vi "自定义DAC.vi"(8 "Vref V":dbl=2.56, 11 "数字编码":dbl[](array[numeric])) -> (2 "输出 V":dbl)   [LabVIEW 2020]
uses:
  <vilib>/express/express arith-compare/Formula/XNode/ExpressFormulaBlockNode.xnode
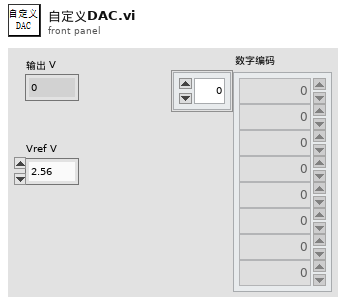
[diagram p1: front panel]
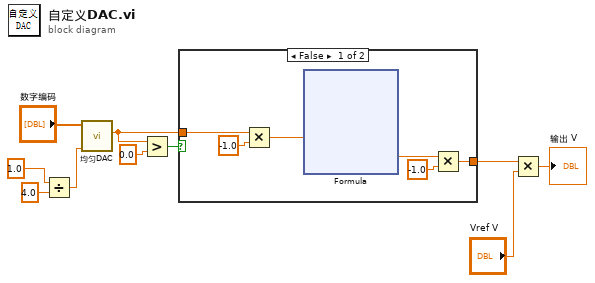
[diagram p0: block diagram]
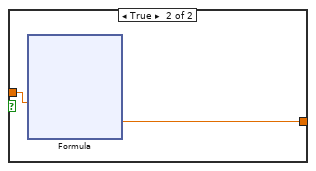
[diagram p2: hidden frame]
diagram:
  n1 = Divide(x=1.0, y=4.0) -> (x/y=w7:dbl)
  n2 = call "均匀DAC.vi"("量化阶 V"=w7, "数字编码"="数字编码") -> ("x+y"=w4:dbl)  [unwired: 9 in]
  n3 = Greater?(x=w4, y=0.0) -> (0:w5:bool)
  n4 = case shown="False" w5 {
    tunnel: w4 -> [w16 w26]
    tunnel: [w12 w25] -> w2
    frame False {
      n5 = Multiply(x=w16, y=-1.0) -> (x*y=w14:dbl)
      n6 = xnode "Formula"("y"=w14) -> ("Result"=w11:dbl)  [unwired: 1 in, 1 out]
      n7 = Multiply(x=w11, y=-1.0) -> (x*y=w12:dbl)
    }
    frame True {
      n8 = xnode "Formula"("y"=w26) -> ("Result"=w25:dbl)  [unwired: 1 in, 1 out]
    }
  }
  n9 = Multiply(x=w2, y="Vref V") -> (x*y=→"输出 V":dbl)
